vi "Query.vi"(8 "error in (no error)":errorcluster, 11 "IMU in":refnum<class "IMU.lvclass">) -> (0 "error out":errorcluster, 2 "Message":string, 3 "IMU out":refnum<class "IMU.lvclass">)   [LabVIEW 2021, in "IMU.lvclass"]
uses:
  IMU.lvclass
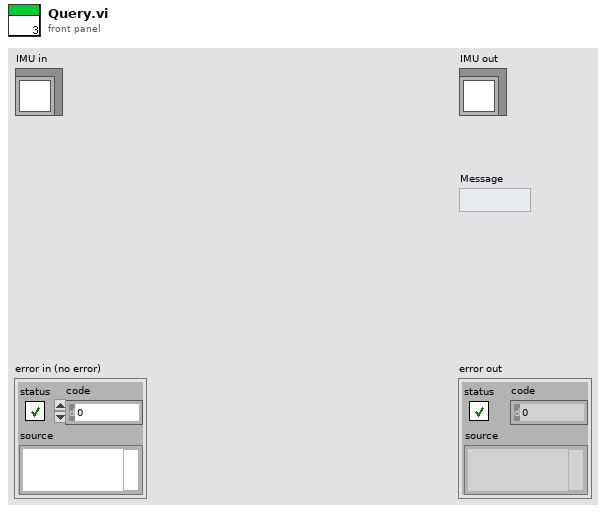
[diagram p1: front panel]
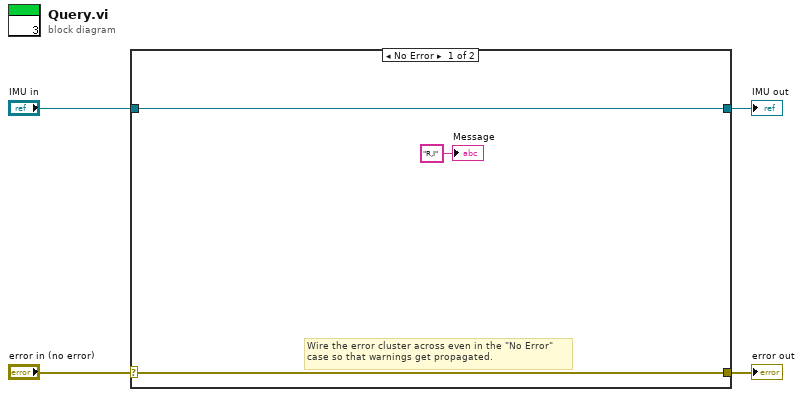
[diagram p0: block diagram]
diagram:
  n1 = case shown="No Error" "error in (no error)" {
    selector: "error in (no error)" -> [w6 w9]
    tunnel: [w6 w9] -> w3
    tunnel: [w7 w8] -> w1
    tunnel: "IMU in" -> [w7 w8]
    frame No Error {
      # "Wire the error cluster across even in the \"No Error\"\ncase so that warnings get propagated."
      "Message" <- "R,I" ("Message")
    }
    frame Error {
    }
  }
  "error out" <- w3
  "IMU out" <- w1
